vi "screen for manual mode entry.vi"() -> ()   [LabVIEW 2022 SP3]
panel:
  in  "?":string
  in  "?":bool
  in  "?":bool
  in  "Close Button":bool
  in  "Begin Manual Job":bool
  # "START NEW\nOPERATION"
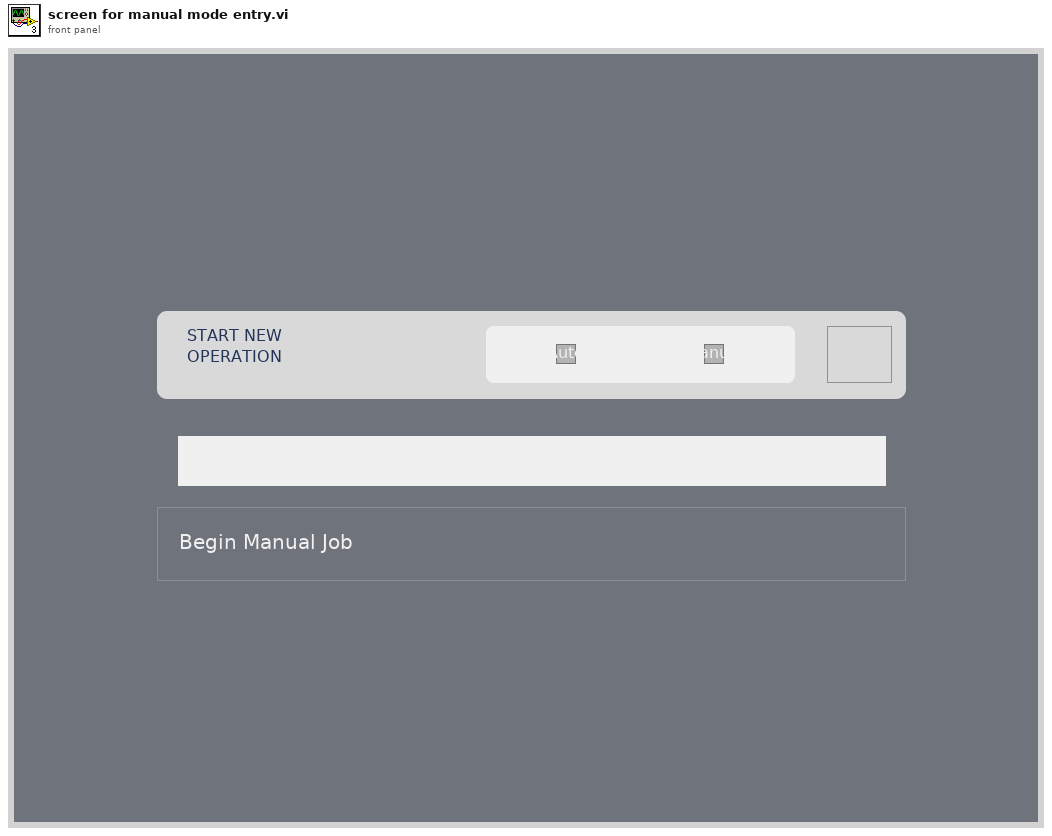
[diagram p1: front panel]
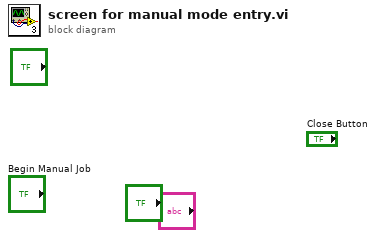
[diagram p0: block diagram]
diagram:
